vi "Segway - Segue objeto 2 controladores.vi"() -> ()   [LabVIEW 2016]
uses:
  <vilib>/NXT/Block Support/NXT_InputPort.ctl
  <vilib>/NXT/Subs/MotorOutput.ctl
  <vilib>/NXT/Block Support/NXT_TimerIndex.ctl
  <vilib>/NXT/Block Support/NXT_OutputPort.ctl
  <vilib>/NXT/Dual Mode Library/Waits/Wait_Num.vi
  <vilib>/NXT/Dual Mode Library/Sensors/EV3_Gyro_Reset.vi
  <vilib>/NXT/Dual Mode Library/Motors/ResetMotor.vi
  <vilib>/NXT/Dual Mode Library/Sensors/EV3_Ultrasonic_CM.vi
  <vilib>/NXT/Dual Mode Library/Display/drawNumber.vi
  <vilib>/NXT/Dual Mode Library/Sensors/EV3_Gyro_Rate.vi
  <vilib>/NXT/Dual Mode Library/Motors/Rotation.vi
  <vilib>/NXT/NXTIO Xnodes/NXTIONodeSubVIs/NXTMoveMotors.vi
  <vilib>/NXT/NXTIO Xnodes/AddressXNode/NXTIOAddress.xnode
  <vilib>/NXT/NXTIO Xnodes/NXTIOXNode/NXTIO.xnode
  <vilib>/NXT/Subs/LVHSConnector.ctl
  <vilib>/NXT/LegoClasses/BrickReference/BrickReference.lvclass
panel:
  in  "stop":bool
  out "e":dbl
  out "Waveform Chart 2":dbl(graph)
  out "b":dbl
  out "a":dbl
  in  "dt_program_flow":dbl
  out "dt":dbl
  out "timer_time":dbl
  out "EncSum":dbl
  out "VelAngRoda2":dbl(graph)
  out "PosAngRoda2":dbl(graph)
  out "PosAngCorpo2":dbl(graph)
  out "VelAngCorpo2":dbl(graph)
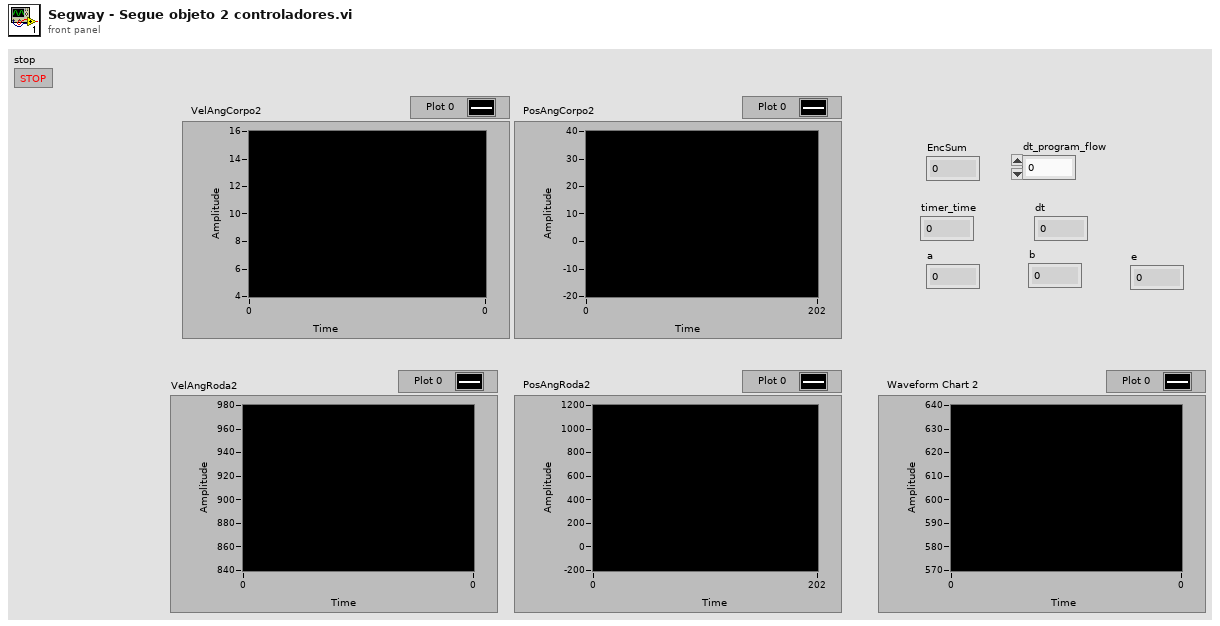
[diagram p1: front panel]
types:
  T1 = typedef "NXT_TimerIndex.ctl" = u8
  T2 = typedef "MotorOutput.ctl" = u8
  T3 = typedef "NXT_InputPort.ctl" = u32
  T4 = typedef "LVHSConnector.ctl" = refnum<class "BrickReference.lvclass">
  T5 = typedef "NXT_OutputPort.ctl" = u8
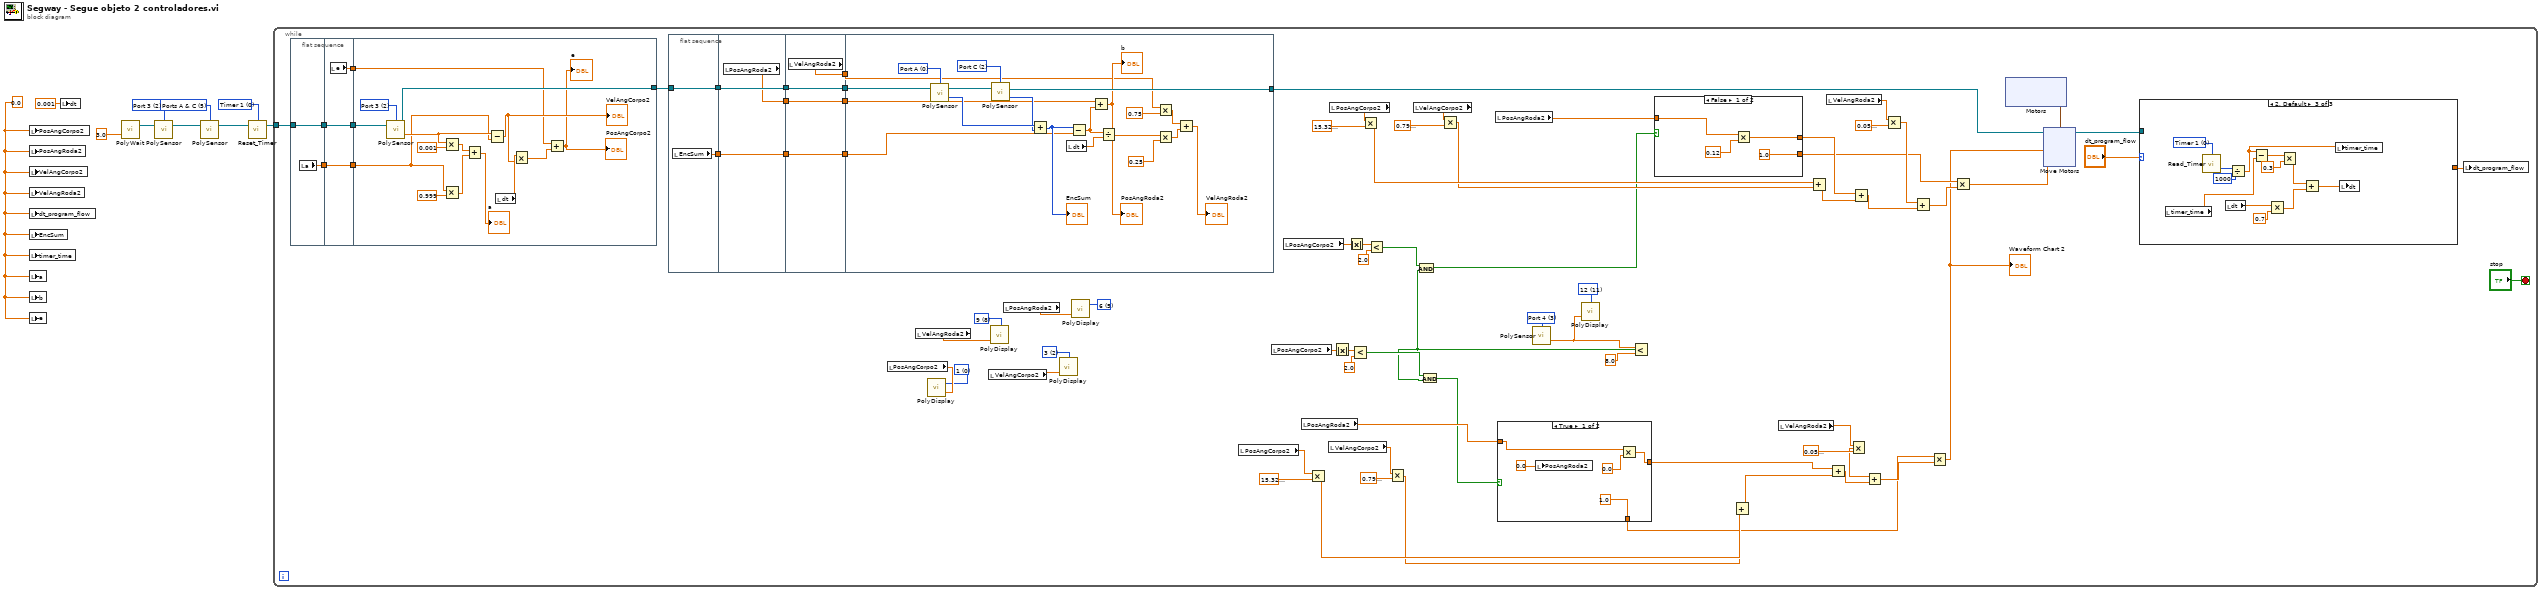
[diagram p0: block diagram]
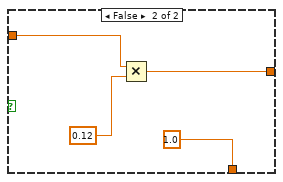
[diagram p2: hidden frame]
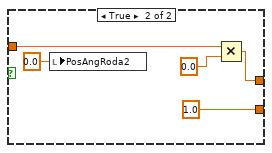
[diagram p3: hidden frame]
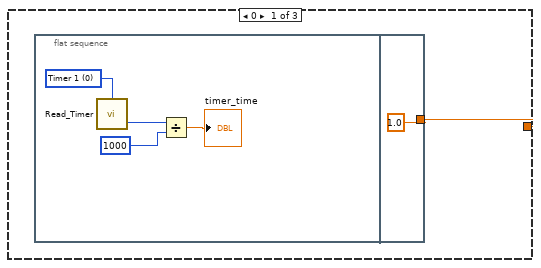
[diagram p4: hidden frame]
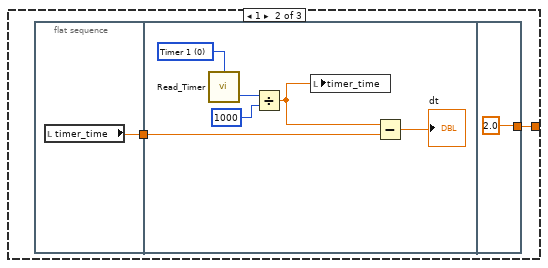
[diagram p5: hidden frame]
diagram:
  w3 = T1 0 items=["Timer 1", "Timer 2", "Timer 3"] ("Timer (Timer 1)")
  w8 = T2 5 items=["Port A"=0, "Port B"=1, "Port C"=2, "Ports A & B"=4, "Ports A & C"=5, "Ports B & C"=6, "All Ports"=3] ("Port (All Ports)")
  w9 = T3 2 items=["Port 1", "Port 2", "Port 3", "Port 4"] ("Port (Port 1)")
  w5 = 0.0 ("PosAngCorpo2")
  n1 = local write "PosAngCorpo2"(w5) -> ()
  n2 = local write "PosAngRoda2"(w5) -> ()
  n3 = local write "VelAngCorpo2"(w5) -> ()
  n4 = local write "VelAngRoda2"(w5) -> ()
  n5 = local write "dt_program_flow"(w5) -> ()
  n6 = local write "EncSum"(w5) -> ()
  n7 = local write "timer_time"(w5) -> ()
  n8 = local write "a"(w5) -> ()
  n9 = local write "b"(w5) -> ()
  n10 = local write "e"(w5) -> ()
  n11 = local write "dt"(0.001 ("dt")) -> ()
  n12 = call-poly <vilib>:"PolyWait.vi"("Time (1 sec)"=sgl 3.0) -> ("NXT/EV3"=w4:T4)  [unwired: 3 in]
  n13 = call-poly <vilib>:"PolySensor.vi"("NXT/EV3"=w4, "Port (Port 1)"=w9) -> ("NXT/EV3"=w7:T4)  [unwired: 2 in]
  n14 = call-poly <vilib>:"PolySensor.vi"("NXT/EV3"=w7, "Port (All Ports)"=w8) -> ("NXT/EV3"=w1:T4)  [unwired: 2 in]
  n15 = call <vilib>:"Reset_Timer.vi"("NXT/EV3"=w1, "Timer (Timer 1)"=w3) -> ("NXT/EV3"=w2:T4)  [unwired: 2 in]
  n16 = while {
    tunnel: w2 -> [w75]
    stop <- "stop" stop-if-true
    w14 = i16 11 items=["1", "2", "3", "4", "5", "6", "7", "8", "9", "10", "11", "12"] ("Line")
    w19 = T3 3 items=["Port 1", "Port 2", "Port 3", "Port 4"] ("Port (Port 1)")
    w50 = i16 5 items=["1", "2", "3", "4", "5", "6", "7", "8", "9", "10", "11", "12"] ("Line")
    w51 = i16 8 items=["1", "2", "3", "4", "5", "6", "7", "8", "9", "10", "11", "12"] ("Line")
    w52 = i16 2 items=["1", "2", "3", "4", "5", "6", "7", "8", "9", "10", "11", "12"] ("Line")
    w54 = i16 0 items=["1", "2", "3", "4", "5", "6", "7", "8", "9", "10", "11", "12"] ("Line")
    n17 = flat-sequence {
      tunnel: w75 -> [w136]
      tunnel: [w136] -> w69
      tunnel: [w135] -> w67
      tunnel: w69 -> [w139]
      tunnel: [w139] -> w68
      tunnel: w67 -> [w138]
      tunnel: [w138] -> w66
      tunnel: [w137] -> w65
      tunnel: [w146] -> w78
      tunnel: w68 -> [w142]
      tunnel: w66 -> [w141]
      tunnel: w65 -> [w140]
      frame #0 {
        n18 = local read "a"() -> (w135:dbl)
      }
      frame #1 {
        n19 = local read "e"() -> (w137:dbl)
      }
      frame #2 {
        w150 = T3 2 items=["Port 1", "Port 2", "Port 3", "Port 4"] ("Port (Port 1)")
        n20 = call-poly <vilib>:"PolySensor.vi"("NXT/EV3"=w142, "Port (Port 1)"=w150) -> ("Degrees/Second"=w149:sgl, "NXT/EV3"=w146:T4)  [unwired: 1 in]
        n21 = Multiply(x=w149, y=0.001) -> (x*y=w152:dbl)
        n22 = Multiply(x=w141, y=0.999) -> (x*y=w145:dbl)
        n23 = Add(x=w152, y=w145) -> (x+y=→"a":dbl)
        n24 = Subtract(x=w149, y=w141) -> (x-y=w147:dbl)
        "VelAngCorpo2" <- w147
        n25 = local read "dt"() -> (w148:dbl)
        n26 = Multiply(x=w148, y=w147) -> (x*y=w151:dbl)
        n27 = Add(x=w140, y=w151) -> (x+y=→"PosAngCorpo2" →"e":dbl)
      }
    }
    n28 = flat-sequence {
      tunnel: w78 -> [w107]
      tunnel: [w107] -> w64
      tunnel: [w106] -> w63
      tunnel: w64 -> [w110]
      tunnel: [w110] -> w62
      tunnel: w63 -> [w109]
      tunnel: [w109] -> w60
      tunnel: [w108] -> w57
      tunnel: w62 -> [w114]
      tunnel: [w114] -> w61
      tunnel: w60 -> [w113]
      tunnel: [w113] -> w59
      tunnel: [w112] -> w58
      tunnel: w57 -> [w111]
      tunnel: [w111] -> w56
      tunnel: w61 -> [w123]
      tunnel: [w121] -> w77
      tunnel: w59 -> [w117]
      tunnel: w58 -> [w116]
      tunnel: w56 -> [w115]
      frame #0 {
        n29 = local read "EncSum"() -> (w106:dbl)
      }
      frame #1 {
        n30 = local read "PosAngRoda2"() -> (w108:dbl)
      }
      frame #2 {
        n31 = local read "VelAngRoda2"() -> (w112:dbl)
      }
      frame #3 {
        w125 = T5 2 items=["Port A", "Port B", "Port C", "Port D"] ("Port (Port A)")
        w128 = T5 0 items=["Port A", "Port B", "Port C", "Port D"] ("Port (Port A)")
        n32 = call-poly <vilib>:"PolySensor.vi"("NXT/EV3"=w123, "Port (Port A)"=w128) -> ("Angle of Rotation"=w127:i32, "NXT/EV3"=w122:T4)  [unwired: 1 in]
        n33 = call-poly <vilib>:"PolySensor.vi"("NXT/EV3"=w122, "Port (Port A)"=w125) -> ("Angle of Rotation"=w124:i32, "NXT/EV3"=w121:T4)  [unwired: 1 in]
        n34 = Add(x=w127, y=w124) -> (x+y=w134:i32)
        "EncSum" <- w134
        n35 = local read "dt"() -> (w126:dbl)
        n36 = Subtract(x=w134, y=w117) -> (x-y=w133:dbl)
        n37 = Add(x=w115, y=w133) -> (x+y=→"PosAngRoda2" →"b":dbl)
        n38 = Divide(x=w133, y=w126) -> (x/y=w129:dbl)
        n39 = Multiply(x=w116, y=0.75) -> (x*y=w119:dbl)
        n40 = Multiply(x=w129, y=sgl 0.25) -> (x*y=w131:dbl)
        n41 = Add(x=w119, y=w131) -> (x+y=→"VelAngRoda2":dbl)
      }
    }
    n42 = local read "PosAngCorpo2"() -> (w55:dbl)
    n43 = local read "VelAngRoda2"() -> (w48:dbl)
    n44 = call-poly <vilib>:"PolyDisplay.vi"("number"=w55, "Line"=w54) -> ()  [unwired: 2 in, 1 out]
    n45 = local read "VelAngCorpo2"() -> (w53:dbl)
    n46 = call-poly <vilib>:"PolyDisplay.vi"("number"=w48, "Line"=w51) -> ()  [unwired: 2 in, 1 out]
    n47 = local read "PosAngRoda2"() -> (w49:dbl)
    n48 = call-poly <vilib>:"PolyDisplay.vi"("number"=w53, "Line"=w52) -> ()  [unwired: 2 in, 1 out]
    n49 = call-poly <vilib>:"PolyDisplay.vi"("number"=w49, "Line"=w50) -> ()  [unwired: 2 in, 1 out]
    n50 = local read "PosAngCorpo2"() -> (w28:dbl)
    n51 = local read "PosAngCorpo2"() -> (w21:dbl)
    n52 = local read "PosAngCorpo2"() -> (w20:dbl)
    n53 = local read "PosAngRoda2"() -> (w26:dbl)
    n54 = Multiply(x=w28, y=sgl 15.33) -> (x*y=w37:dbl)
    n55 = local read "VelAngCorpo2"() -> (w29:dbl)
    n56 = local read "PosAngCorpo2"() -> (w81:dbl)
    n57 = Absolute Value(x=w21) -> (abs(x)=w30:dbl)
    n58 = Absolute Value(x=w20) -> (abs(x)=w41:dbl)
    n59 = Less?(x=w30, y=2.0) -> (x < y?=w13:bool)
    n60 = Multiply(x=w81, y=sgl 15.33) -> (x*y=w74:dbl)
    n61 = Less?(x=w41, y=2.0) -> (x < y?=w12:bool)
    n62 = Multiply(x=w29, y=sgl 0.79) -> (x*y=w36:dbl)
    n63 = local read "VelAngCorpo2"() -> (w80:dbl)
    n64 = Multiply(x=w80, y=sgl 0.79) -> (x*y=w73:dbl)
    n65 = local read "PosAngRoda2"() -> (w45:dbl)
    n66 = call-poly <vilib>:"PolySensor.vi"("Port (Port 1)"=w19) -> ("Centimeters"=w15:sgl)  [unwired: 2 in, 1 out]
    n67 = call-poly <vilib>:"PolyDisplay.vi"("number"=w15, "Line"=w14) -> ()  [unwired: 2 in, 1 out]
    n68 = Less?(x=w15, y=8.0) -> (x < y?=w11:bool)
    n69 = And(x=w12, y=w11) -> (x .and. y?=w17:bool)
    n70 = And(x=w13, y=w11) -> (x .and. y?=w16:bool)
    n71 = case shown="True" w16 {
      tunnel: w26 -> [w90 w95]
      tunnel: [w89 w94] -> w25
      tunnel: [1.0 1.0 ("y")] -> w24
      frame True {
        n72 = local write "PosAngRoda2"(0.0) -> ()
        n73 = Multiply(x=w90, y=0.0) -> (x*y=w89:dbl)
      }
      frame False {
        n74 = Multiply(x=w95, y=0.12) -> (x*y=w94:dbl)
      }
    }
    n75 = case shown="False" w17 {
      tunnel: w45 -> [w100 w104]
      tunnel: [w98 w103] -> w44
      tunnel: [1.0 ("y") 1.0 ("y")] -> w43
      frame False {
        n76 = Multiply(x=w100, y=0.12) -> (x*y=w98:dbl)
      }
      frame True {
        n77 = local write "PosAngRoda2"(0.0 ("PosAngRoda2")) -> ()
        n78 = Multiply(x=w104, y=0.0) -> (x*y=w103:dbl)
      }
    }
    n79 = Add(x=w37, y=w36) -> (x+y=w35:dbl)
    n80 = local read "VelAngRoda2"() -> (w27:dbl)
    n81 = Add(x=w74, y=w73) -> (x+y=w72:dbl)
    n82 = local read "VelAngRoda2"() -> (w79:dbl)
    n83 = Add(x=w25, y=w35) -> (x+y=w34:dbl)
    n84 = Multiply(x=w27, y=sgl 0.06) -> (x*y=w33:dbl)
    n85 = Add(x=w44, y=w72) -> (x+y=w71:dbl)
    n86 = Add(x=w33, y=w34) -> (x+y=w31:dbl)
    n87 = Multiply(x=w79, y=sgl 0.06) -> (x*y=w70:dbl)
    n88 = Add(x=w70, y=w71) -> (x+y=w42:dbl)
    n89 = Multiply(x=w24, y=w31) -> (x*y=w22:dbl)
    "Waveform Chart 2" <- w22
    n90 = Multiply(x=w43, y=w42) -> (x*y=w23:dbl)
    n91 = xnode "Motors"() -> ("Motor"=w85:cluster{"Port":T5, "Port":T5})
    n92 = xnode "Move Motors"("Power/Speed 2"=w22, "Power/Speed 1"=w23, "Motors"=w85, "NXT/EV3"=w77) -> ("NXT/EV3"=w76:T4)
    n93 = case shown="2, Default" "dt_program_flow" {
      tunnel: [w164 w170 _] -> w87
      tunnel: w76 -> [_ _ _]
      frame 0 {
        n94 = flat-sequence {
          tunnel: [1.0 ("dt_program_flow")] -> w164
          frame #0 {
            w168 = T1 0 items=["Timer 1", "Timer 2", "Timer 3"] ("Timer (Timer 1)")
            n95 = call <vilib>:"Read_Timer.vi"("Timer (Timer 1)"=w168) -> ("Value (msec)"=w165:u32)  [unwired: 2 in, 1 out]
            n96 = Divide(x=w165, y=u32 1000) -> (x/y=→"timer_time":dbl)
          }
          frame #1 {
          }
        }
      }
      frame 1 {
        n97 = flat-sequence {
          tunnel: [w172] -> w171
          tunnel: w171 -> [w178]
          tunnel: [2.0 ("dt_program_flow")] -> w170
          frame #0 {
            n98 = local read "timer_time"() -> (w172:dbl)
          }
          frame #1 {
            w176 = T1 0 items=["Timer 1", "Timer 2", "Timer 3"] ("Timer (Timer 1)")
            n99 = call <vilib>:"Read_Timer.vi"("Timer (Timer 1)"=w176) -> ("Value (msec)"=w175:u32)  [unwired: 2 in, 1 out]
            n100 = Divide(x=w175, y=u32 1000) -> (x/y=w173:dbl)
            n101 = local write "timer_time"(w173) -> ()
            n102 = Subtract(x=w173, y=w178) -> (x-y=→"dt":dbl)
          }
          frame #2 {
          }
        }
      }
      frame 2, Default {
        w183 = T1 0 items=["Timer 1", "Timer 2", "Timer 3"] ("Timer (Timer 1)")
        n103 = local read "timer_time"() -> (w180:dbl)
        n104 = call <vilib>:"Read_Timer.vi"("Timer (Timer 1)"=w183) -> ("Value (msec)"=w182:u32)  [unwired: 2 in, 1 out]
        n105 = local read "dt"() -> (w185:dbl)
        n106 = Divide(x=w182, y=u32 1000) -> (x/y=w190:dbl)
        n107 = Subtract(x=w190, y=w180) -> (x-y=w189:dbl)
        n108 = Multiply(x=w185, y=0.7) -> (x*y=w184:dbl)
        n109 = Multiply(x=w189, y=0.3) -> (x*y=w187:dbl)
        n110 = Add(x=w187, y=w184) -> (x+y=w191:dbl)
        n111 = local write "timer_time"(w190) -> ()
        n112 = local write "dt"(w191) -> ()
      }
    }
    n113 = local write "dt_program_flow"(w87) -> ()
  }
